vi "Update.vi"(8 "error in (no error)":errorcluster, 10 "Message in":refnum<class "UpdateMessage.lvclass">, 11 "ImageStack in":refnum<class "ImageStack.lvclass">) -> (0 "error out":errorcluster, 3 "ImageStack out":refnum<class "ImageStack.lvclass">)   [LabVIEW 2012, in "ImageStack.lvclass"]
doc: "The update method processes the command 'update'. \n\nThe command 'update' is used for receiving new values to be set to the private data of the class. This could be seen as a public set method for setting new parameters to the private class data."
uses:
  ImageStack.lvclass
  <vilib>/Distrio/Murmex/UpdateMessage/UpdateMessage.lvclass
  ImageStack.lvclass/ImageStack.ctl
  <vilib>/Distrio/Murmex/Murmex/Murmex.lvclass
panel:
  # "This method is called when the UPDATE\ntrigger is sent. \n\nOverride this method when your component needs to\nrespond to this trigger. \n\nCall parent for proper implementation"
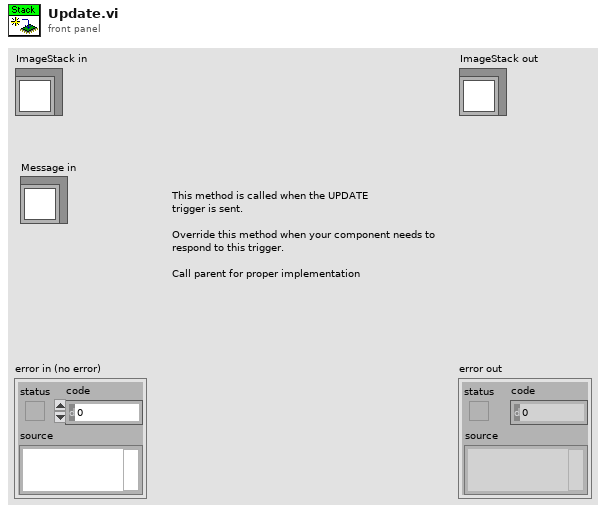
[diagram p1: front panel]
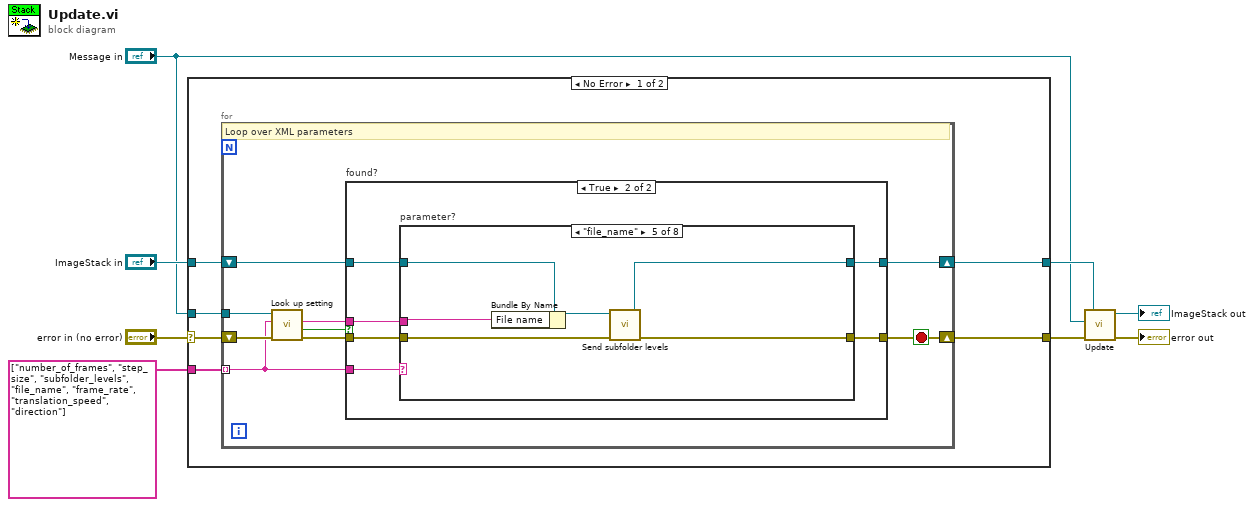
[diagram p0: block diagram]
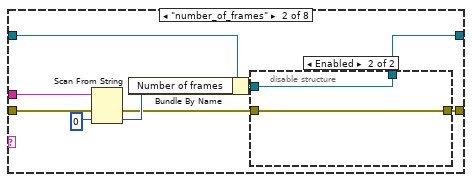
[diagram p4: hidden frame]
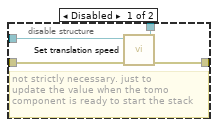
[diagram p5: hidden frame]
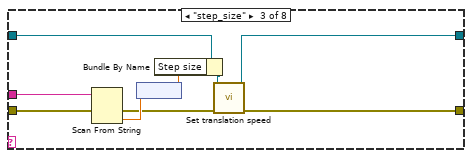
[diagram p6: hidden frame]
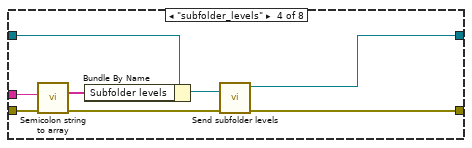
[diagram p7: hidden frame]
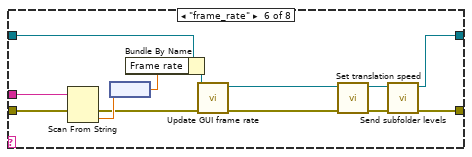
[diagram p8: hidden frame]
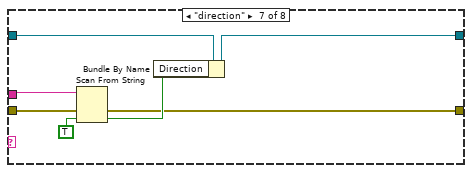
[diagram p9: hidden frame]
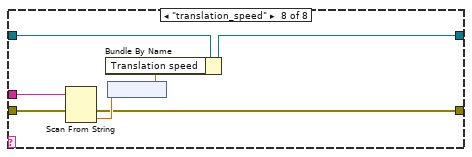
[diagram p10: hidden frame]
diagram:
  n1 = case shown="No Error" "error in (no error)" {
    selector: "error in (no error)" -> [w14 w100]
    tunnel: [w9 w100] -> w1
    tunnel: [w12 w99] -> w6
    tunnel: "ImageStack in" -> [w13 w99]
    tunnel: "Message in" -> [w11 _]
    tunnel: string[] ["number_of_frames", "step_size", "subfolder_levels", "file_name", "frame_rate", "translation_speed", "direction"] -> [w10 _]
    frame No Error {
      n2 = for {
        shift-right: [w15] -> w9
        shift-left: w14 -> [w22]
        shift-right: [w16] -> w12
        shift-left: w13 -> [w18]
        tunnel: w11 -> [w23]
        tunnel: w10 -> [w17] mode=indexing
        stop <- w15 stop-if-true
        # "Loop over XML parameters"
        n3 = call <vilib>:"Look up setting.vi"("error in (no error)"=w22, "tag name"=w17, "UpdateMessage in"=w23) -> ("error out"=w20:errorcluster, "found?"=w21:bool, "value"=w19:string)  [unwired: 5 in, 1 out]
        n4 = case "found?" shown="True" w21 {
          tunnel: w20 -> [w24 w29]
          tunnel: w19 -> [_ w30]
          tunnel: w18 -> [w25 w28]
          tunnel: w17 -> [_ w31]
          tunnel: [w24 w27] -> w15
          tunnel: [w25 w26] -> w16
          frame False {
          }
          frame True {
            n5 = case "parameter?" shown="\"file_name\"" w31 {
              tunnel: w30 -> [_ w42 w57 w64 w70 w80 w89 w93]
              tunnel: w29 -> [w32 w41 w56 w63 w69 w84 w91 w96]
              tunnel: w28 -> [w33 w39 w55 w65 w71 w81 w88 w94]
              tunnel: [w32 w36 w50 w60 w68 w73 w86 w95] -> w27
              tunnel: [w33 w34 w49 w59 w66 w74 w85 w92] -> w26
              frame Default {
              }
              frame "number_of_frames" {
                n6 = Scan From String(input string=w42, error in=w41, default 1=u16 0) -> (error out=w37:errorcluster, output 1=w38:u16)  [unwired: 2 in, 2 out]
                n7 = Bundle By Name(cluster=w39, "Number of frames"=w38) -> (w35:refnum<class "ImageStack.lvclass">)
                n8 = disable-structure shown="Enabled" {
                  disable-tunnel: w37 -> [w46 w47]
                  disable-tunnel: [w45 w47] -> w36
                  disable-tunnel: w35 -> [w44 w48]
                  disable-tunnel: [w43 w48] -> w34
                  frame Disabled {
                    # "not strictly necessary. just to\nupdate the value when the tomo\ncomponent is ready to start the stack"
                    n9 = call-dynamic "Set translation speed.vi"("error in (no error)"=w46, "ImageStack in"=w44) -> ("error out"=w45:errorcluster, "ImageStack out"=w43:refnum<class "ImageStack.lvclass">)  [unwired: 8 in]
                  }
                  frame Enabled {
                  }
                }
              }
              frame "step_size" {
                n10 = Scan From String(input string=w57, error in=w56) -> (error out=w51:errorcluster, output 1=w54:dbl)  [unwired: 3 in, 2 out]
                n11 = node(w54) -> (w53:dbl[unit])
                n12 = Bundle By Name(cluster=w55, "Step size"=w53) -> (w52:refnum<class "ImageStack.lvclass">)
                n13 = call-dynamic "Set translation speed.vi"("error in (no error)"=w51, "ImageStack in"=w52) -> ("error out"=w50:errorcluster, "ImageStack out"=w49:refnum<class "ImageStack.lvclass">)  [unwired: 8 in]
              }
              frame "subfolder_levels" {
                n14 = call "Semicolon string to array.vi"("error in"=w63, "Semicolon string"=w64) -> ("error out"=w61:errorcluster, "String array"=w62:string[])  [unwired: 8 in]
                n15 = Bundle By Name(cluster=w65, "Subfolder levels"=w62) -> (w58:refnum<class "ImageStack.lvclass">)
                n16 = call-dynamic "Send subfolder levels.vi"("error in (no error)"=w61, "ImageStack in"=w58) -> ("error out"=w60:errorcluster, "ImageStack out"=w59:refnum<class "ImageStack.lvclass">)  [unwired: 8 in]
              }
              frame "file_name" {
                n17 = Bundle By Name(cluster=w71, "File name"=w70) -> (w67:refnum<class "ImageStack.lvclass">)
                n18 = call-dynamic "Send subfolder levels.vi"("error in (no error)"=w69, "ImageStack in"=w67) -> ("error out"=w68:errorcluster, "ImageStack out"=w66:refnum<class "ImageStack.lvclass">)  [unwired: 8 in]
              }
              frame "frame_rate" {
                n19 = Scan From String(input string=w80, error in=w84) -> (error out=w79:errorcluster, output 1=w82:dbl)  [unwired: 3 in, 2 out]
                n20 = node(w82) -> (w83:dbl[unit])
                n21 = Bundle By Name(cluster=w81, "Frame rate"=w83) -> (w77:refnum<class "ImageStack.lvclass">)
                n22 = call-dynamic "Update GUI frame rate.vi"("error in (no error)"=w79, "ImageStack in"=w77) -> ("error out"=w78:errorcluster, "ImageStack out"=w76:refnum<class "ImageStack.lvclass">)  [unwired: 8 in]
                n23 = call-dynamic "Set translation speed.vi"("error in (no error)"=w78, "ImageStack in"=w76) -> ("error out"=w72:errorcluster, "ImageStack out"=w75:refnum<class "ImageStack.lvclass">)  [unwired: 8 in]
                n24 = call-dynamic "Send subfolder levels.vi"("error in (no error)"=w72, "ImageStack in"=w75) -> ("error out"=w73:errorcluster, "ImageStack out"=w74:refnum<class "ImageStack.lvclass">)  [unwired: 8 in]
              }
              frame "direction" {
                n25 = Scan From String(input string=w89, error in=w91, default 1=TRUE) -> (error out=w86:errorcluster, output 1=w87:bool)  [unwired: 2 in, 2 out]
                n26 = Bundle By Name(cluster=w88, "Direction"=w87) -> (w85:refnum<class "ImageStack.lvclass">)
              }
              frame "translation_speed" {
                n27 = Scan From String(input string=w93, error in=w96) -> (error out=w95:errorcluster, output 1=w97:dbl)  [unwired: 3 in, 2 out]
                n28 = node(w97) -> (w98:dbl[unit])
                n29 = Bundle By Name(cluster=w94, "Translation speed"=w98) -> (w92:refnum<class "ImageStack.lvclass">)
              }
            }
          }
        }
      }
    }
    frame Error {
    }
  }
  n30 = call-parent "Update.vi"("error in (no error)"=w1, "Message in"="Message in", "Murmex in"=w6) -> ("error out"=→"error out":errorcluster, "Murmex out"=→"ImageStack out":refnum<class "ImageStack.lvclass">)  [unwired: 7 in]
